vi "bee1v2.vi"() -> ()   [LabVIEW 2020]
uses:
  <vilib>/Instr/_visa.llb/VISA Flush IO Buffer Mask.ctl
  <vilib>/Instr/_visa.llb/VISA Configure Serial Port (Instr).vi
  <vilib>/Waveform/DWDTOps.llb/DWDT Boolean Array to Digital.vi
panel:
  in  "start":bool
  in  "stop":bool
  in  "Tab Control":enum32{"Graph", " Config"}(tab)
  out "Digital Waveform Graph":digitalwaveform(graph)
  in  "VISA resource name":refnum<visa-resource-name>
  in  "file path (use dialog)":path
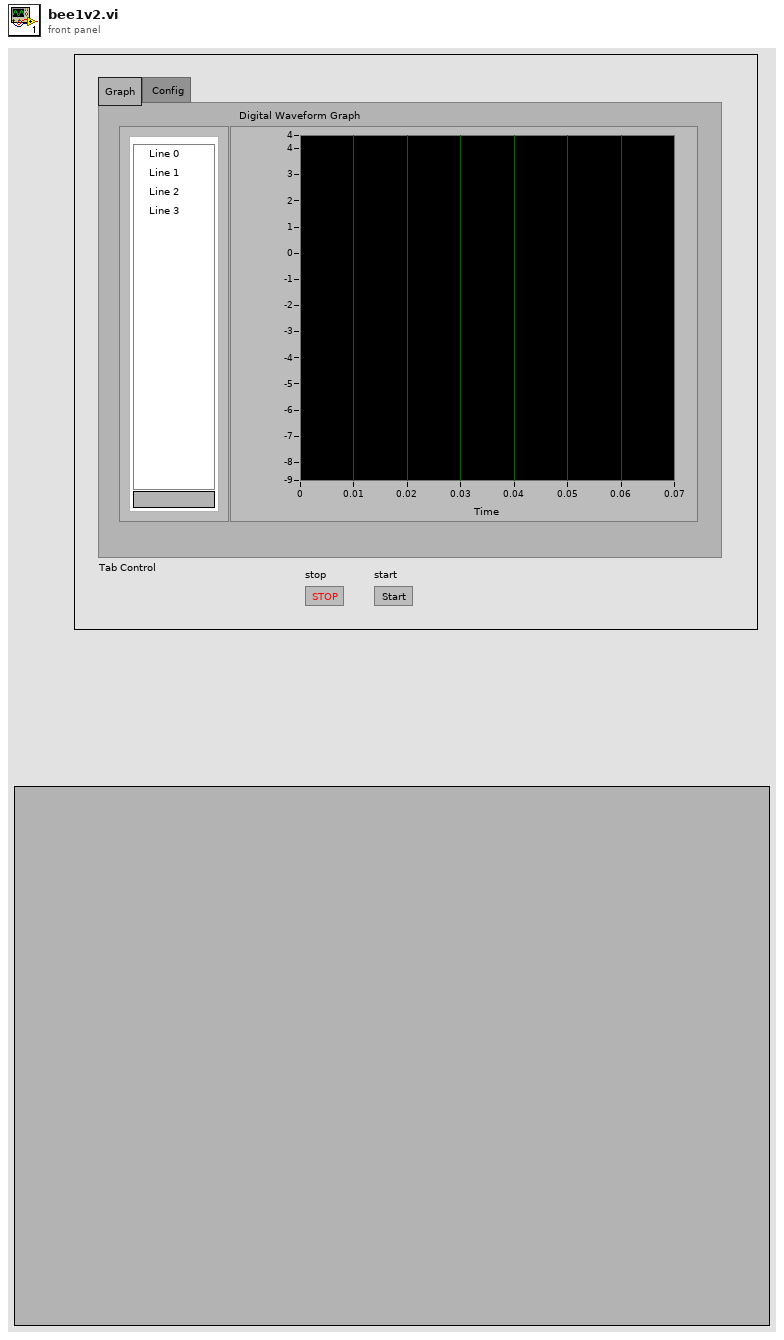
[diagram p1: front panel]
types:
  T1 = enum8{"Enabled", "Disabled", "Disabled and Grayed Out"}
  T2 = enum16{"open", "replace", "create", "open or create", "replace or create", "replace or create with confirmation"}
  T3 = typedef "VISA Flush IO Buffer Mask.ctl" = u16
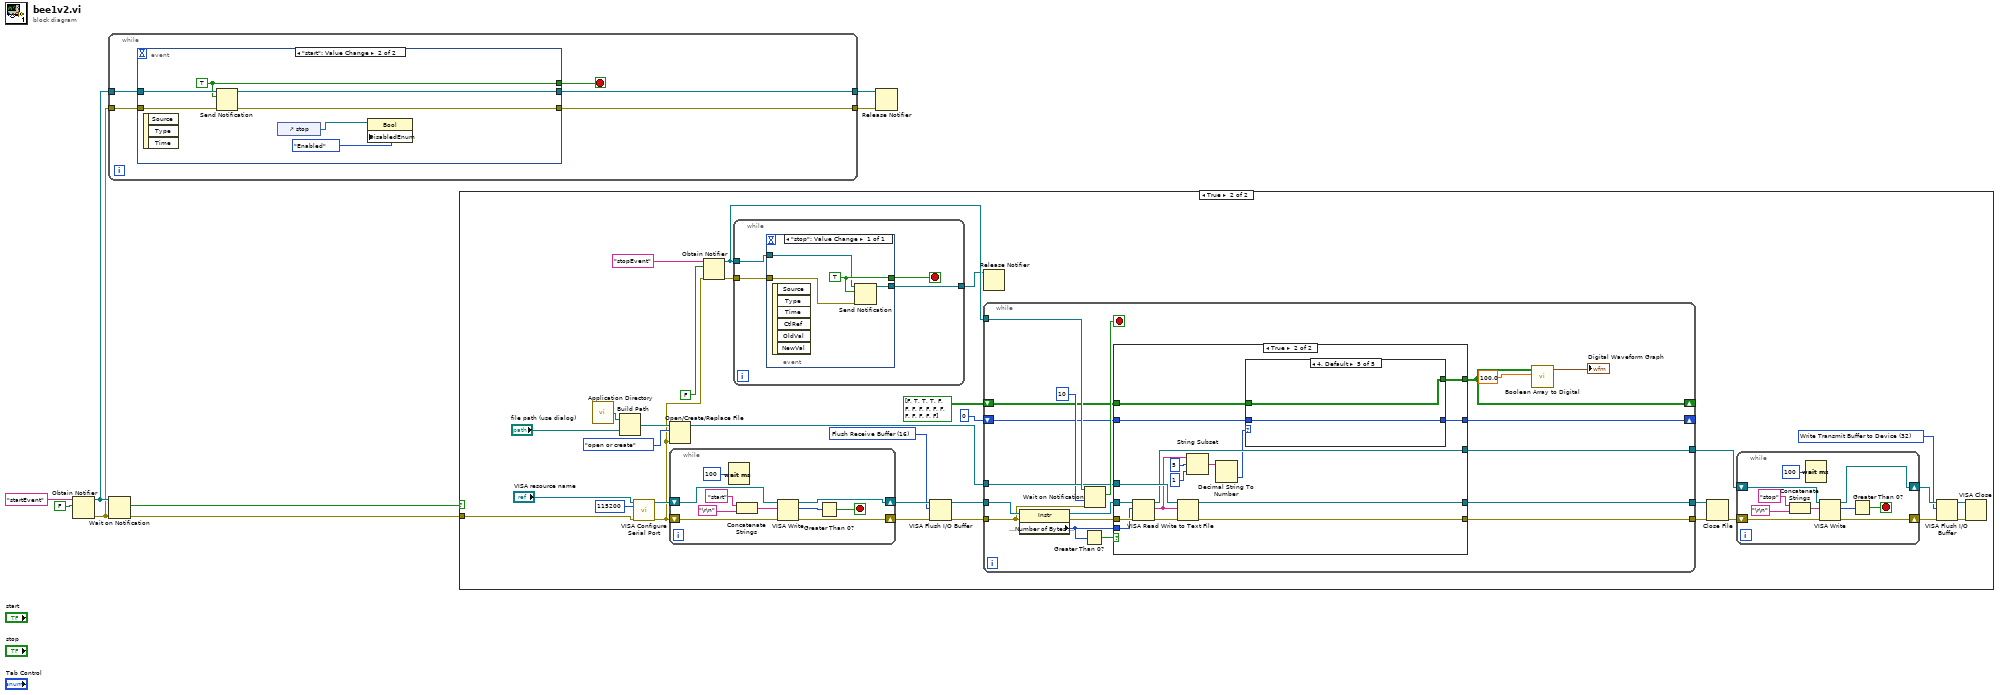
[diagram p0: block diagram]
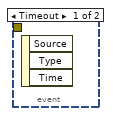
[diagram p2: hidden frame]
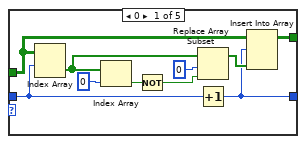
[diagram p5: hidden frame]
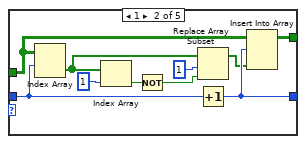
[diagram p6: hidden frame]
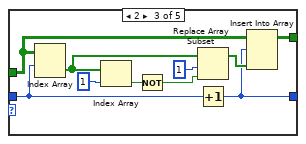
[diagram p7: hidden frame]
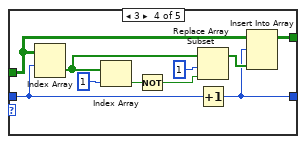
[diagram p8: hidden frame]
diagram:
  n1 = Obtain Notifier(name (unnamed)="startEvent", notification data type=FALSE ("create if not found? (T)")) -> (notifier out=w5:refnum<notifier>, error out=w2:errorcluster)  [unwired: 2 in, 1 out]
  n2 = while {
    tunnel: w5 -> [w13]
    tunnel: [w12] -> w7
    tunnel: w2 -> [w10]
    tunnel: [w9] -> w6
    stop <- w11 stop-if-true
    n3 = event shown="[1] \"start\": Value Change" {
      selector: _ -> [_ _]
      dyn-events: _ -> [_ _]
      timeout: _ -> [_ _]
      tunnel: w13 -> [_ w20]
      tunnel: [_ w19] -> w12
      tunnel: [_ w18] -> w11
      tunnel: w10 -> [_ w17]
      tunnel: [_ w16] -> w9
      event Timeout {
        n4 = event-data() -> ()  [unwired: 1 in, 3 out]
      }
      event "start": Value Change {
        w18 = TRUE
        n5 = event-data() -> ()  [unwired: 1 in, 3 out]
        n6 = Send Notification(notification=w18, notifier=w20, error in (no error)=w17) -> (notifier out=w19:refnum<notifier>, error out=w16:errorcluster)
        n7 = control-ref of="stop"() -> (w15:refnum<vi>)
        n8 = property class="Bool"(reference=w15, "DisabledEnum"=T1."Enabled" ("Disabled")) -> ()  [unwired: 1 in, 2 out]
      }
    }
  }
  n9 = Wait on Notification(notifier=w5, error in (no error)=w2) -> (notification=w4:bool, error out=w1:errorcluster)  [unwired: 2 in, 2 out]
  n10 = case shown="True" w4 {
    tunnel: w1 -> [_ w29]
    frame False {
    }
    frame True {
      w24 = T3 32 items=["Flush Receive Buffer"=16, "Write Transmit Buffer to Device"=32, "Flush Receive Buffer (No I/O)"=64, "Flush Transmit Buffer"=128] ("Mask")
      w30 = T3 16 items=["Flush Receive Buffer"=16, "Write Transmit Buffer to Device"=32, "Flush Receive Buffer (No I/O)"=64, "Flush Transmit Buffer"=128] ("Mask")
      n11 = call <vilib>:"Application Directory.vi"() -> ("Application Directory"=w43:path)
      n12 = Build Path(base path=w43, name or relative path="file path (use dialog)") -> (appended path=w41:path)
      n13 = call-poly "VISA Configure Serial Port"("VISA resource name"="VISA resource name", "baud rate (9600)"=u32 115200, "error in (no error)"=w29) -> ("VISA resource name out"=w39:refnum<visa-resource-name>, "error out"=w35:errorcluster)  [unwired: 11 in]
      n14 = Open/Create/Replace File(file path (use dialog)=w41, error in=w35, operation (0:open)=T2."open or create") -> (refnum out=w44:refnum<file>)  [unwired: 3 in, 2 out]
      n15 = while {
        shift-right: [w63] -> w34
        shift-left: w39 -> [w71]
        shift-right: [w62] -> w33
        shift-left: w35 -> [w70]
        stop <- w69 stop-if-true
        n16 = Wait (ms)(milliseconds to wait=u32 100) -> ()  [unwired: 1 out]
        n17 = Concatenate Strings("start" ("write buffer"), "\r\n") -> (w64:string)
        n18 = VISA Write(VISA resource name=w71, write buffer=w64, error in (no error)=w70) -> (VISA resource name out=w63:refnum<visa-resource-name>, return count=w68:u32, error out=w62:errorcluster)
        n19 = Greater Than 0?(x=w68) -> (x > 0?=w69:bool)
      }
      n20 = Obtain Notifier(name (unnamed)="stopEvent", notification data type=FALSE, error in (no error)=w35) -> (notifier out=w49:refnum<notifier>, error out=w46:errorcluster)  [unwired: 1 in, 1 out]
      n21 = while {
        tunnel: w49 -> [w74]
        tunnel: [w72] -> w48
        tunnel: w46 -> [w73]
        stop <- w75 stop-if-true
        n22 = event shown="[0] \"stop\": Value Change" {
          selector: _ -> [_]
          dyn-events: _ -> [_]
          timeout: _ -> [_]
          tunnel: [w79] -> w75
          tunnel: w74 -> [w78]
          tunnel: w73 -> [w77]
          tunnel: [w76] -> w72
          event "stop": Value Change {
            w79 = TRUE
            n23 = event-data() -> ()  [unwired: 1 in, 6 out]
            n24 = Send Notification(notification=w79, notifier=w78, error in (no error)=w77) -> (notifier out=w76:refnum<notifier>)  [unwired: 1 out]
          }
        }
      }
      n25 = VISA Flush I/O Buffer(VISA resource name=w34, mask (16)=w30, error in (no error)=w33) -> (VISA resource name out=w32:refnum<visa-resource-name>, error out=w31:errorcluster)
      n26 = Release Notifier(notifier=w48) -> ()  [unwired: 2 in, 3 out]
      n27 = while {
        tunnel: w49 -> [w98]
        tunnel: w32 -> [w96]
        tunnel: w31 -> [w85]
        tunnel: w44 -> [w91]
        tunnel: [w90] -> w22
        tunnel: [w89] -> w23
        tunnel: [w88] -> w38
        shift-right: [w80] -> _
        shift-left: bool[][] [[FALSE, TRUE, TRUE, TRUE], [FALSE, FALSE, FALSE, FALSE], [FALSE, FALSE, FALSE, FALSE], [FALSE, FALSE, FALSE, FALSE]] -> [w83]
        shift-right: [w81] -> _
        shift-left: 0 -> [w82]
        stop <- w97 stop-if-true
        n28 = property class="Instr"(reference=w96, error in=w85) -> (reference out=w94:refnum<visa-resource-name>, error out=w95:errorcluster, "Serial Settings:Number of Bytes at Serial Port"=w92:u32)
        n29 = Greater Than 0?(x=w92) -> (x > 0?=w93:bool)
        n30 = Wait on Notification(notifier=w98, timeout in ms (-1)=10, error in (no error)=w85) -> (notification=w97:bool)  [unwired: 1 in, 3 out]
        n31 = case shown="True" w93 {
          tunnel: w95 -> [w102 w120]
          tunnel: w94 -> [w101 w119]
          tunnel: w92 -> [_ w118]
          tunnel: w91 -> [w103 w117]
          tunnel: [w103 w115] -> w90
          tunnel: [w102 w114] -> w89
          tunnel: [w101 w113] -> w88
          tunnel: [w100 w107] -> w80
          tunnel: w83 -> [w100 w106]
          tunnel: w82 -> [w99 w105]
          tunnel: [w99 w104] -> w81
          frame False {
          }
          frame True {
            n32 = VISA Read(VISA resource name=w119, byte count=w118, error in (no error)=w120) -> (VISA resource name out=w113:refnum<visa-resource-name>, read buffer=w108:string, error out=w116:errorcluster)  [unwired: 1 out]
            n33 = Write to Text File(file (use dialog)=w117, text=w108, error in=w116) -> (refnum out=w115:refnum<file>, error out=w114:errorcluster)  [unwired: 1 in, 1 out]
            n34 = String Subset(string=w108, offset (0)=5, length (rest)=1 ("length (rest)")) -> (substring=w110:string)
            n35 = Decimal String To Number(string=w110) -> (number=w109:i32)  [unwired: 2 in, 1 out]
            n36 = case shown="4, Default" w109 {
              tunnel: [w123 w140 w143 w154 w162] -> w107
              tunnel: w106 -> [w124 w137 w142 w151 w162]
              tunnel: w105 -> [w121 w139 w141 w152 w161]
              tunnel: [w122 w138 w144 w153 w161] -> w104
              frame 0 {
                n37 = Index Array(array=w124, index (row)=w121) -> (element=w127:bool[])  [unwired: 1 in]
                n38 = Index Array(array=w127, index=0) -> (element=w130:bool)
                n39 = Not(x=w130) -> (.not. x?=w129:bool)
                n40 = Replace Array Subset(array=w127, new element=w129, index=0) -> (w128:bool[])
                n41 = Increment(x=w121) -> (x+1=w122:i32)
                n42 = Insert Into Array(array=w124, index (row)=w122, new element=w128) -> (w123:bool[][])  [unwired: 1 in]
              }
              frame 1 {
                n43 = Index Array(array=w137, index (row)=w139) -> (element=w135:bool[])  [unwired: 1 in]
                n44 = Index Array(array=w135, index=1) -> (element=w131:bool)
                n45 = Not(x=w131) -> (.not. x?=w132:bool)
                n46 = Replace Array Subset(array=w135, new element=w132, index=1) -> (w133:bool[])
                n47 = Increment(x=w139) -> (x+1=w138:i32)
                n48 = Insert Into Array(array=w137, index (row)=w138, new element=w133) -> (w140:bool[][])  [unwired: 1 in]
              }
              frame 2 {
                n49 = Index Array(array=w142, index (row)=w141) -> (element=w147:bool[])  [unwired: 1 in]
                n50 = Index Array(array=w147, index=1) -> (element=w150:bool)
                n51 = Not(x=w150) -> (.not. x?=w149:bool)
                n52 = Replace Array Subset(array=w147, new element=w149, index=1) -> (w148:bool[])
                n53 = Increment(x=w141) -> (x+1=w144:i32)
                n54 = Insert Into Array(array=w142, index (row)=w144, new element=w148) -> (w143:bool[][])  [unwired: 1 in]
              }
              frame 3 {
                n55 = Index Array(array=w151, index (row)=w152) -> (element=w159:bool[])  [unwired: 1 in]
                n56 = Index Array(array=w159, index=1) -> (element=w155:bool)
                n57 = Not(x=w155) -> (.not. x?=w156:bool)
                n58 = Replace Array Subset(array=w159, new element=w156, index=1) -> (w157:bool[])
                n59 = Increment(x=w152) -> (x+1=w153:i32)
                n60 = Insert Into Array(array=w151, index (row)=w153, new element=w157) -> (w154:bool[][])  [unwired: 1 in]
              }
              frame 4, Default {
              }
            }
          }
        }
        n61 = call-poly <vilib>:"Boolean Array to Digital.vi"("sample rate"=100.0, "boolean array"=w80) -> ("digital waveform"=→"Digital Waveform Graph":digitalwaveform)  [unwired: 8 in, 1 out]
      }
      n62 = Close File(refnum=w22, error in=w23) -> (error out=w21:errorcluster)  [unwired: 1 out]
      n63 = while {
        shift-right: [w56] -> w27
        shift-left: w21 -> [w55]
        shift-right: [w57] -> w28
        shift-left: w38 -> [w61]
        stop <- w53 stop-if-true
        n64 = Concatenate Strings("stop" ("write buffer"), "\r\n") -> (w58:string)
        n65 = Wait (ms)(milliseconds to wait=u32 100) -> ()  [unwired: 1 out]
        n66 = VISA Write(VISA resource name=w61, write buffer=w58, error in (no error)=w55) -> (VISA resource name out=w57:refnum<visa-resource-name>, return count=w54:u32, error out=w56:errorcluster)
        n67 = Greater Than 0?(x=w54) -> (x > 0?=w53:bool)
      }
      n68 = VISA Flush I/O Buffer(VISA resource name=w28, mask (16)=w24, error in (no error)=w27) -> (VISA resource name out=w25:refnum<visa-resource-name>, error out=w26:errorcluster)
      n69 = VISA Close(VISA resource name=w25, error in (no error)=w26) -> ()  [unwired: 1 out]
    }
  }
  n70 = Release Notifier(notifier=w7, error in (no error)=w6) -> ()  [unwired: 1 in, 3 out]
